vi "ClimberDeploy.vi"(8 "error in (no error)":errorcluster, 9 "Deploy":bool, 10 "Screw":dbl, 11 "Climber in":refnum<class "Climber.lvclass">) -> (0 "error out":errorcluster, 3 "Climber out":refnum<class "Climber.lvclass">)   [LabVIEW 2019, in "Climber.lvlib" / "Climber.lvclass"]
uses:
  Climber.lvclass
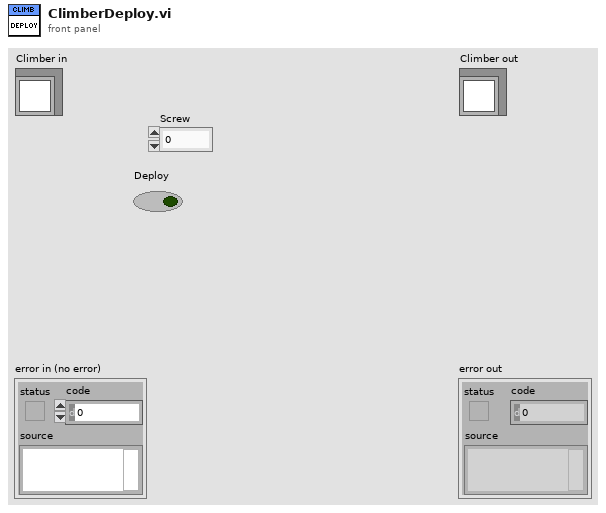
[diagram p1: front panel]
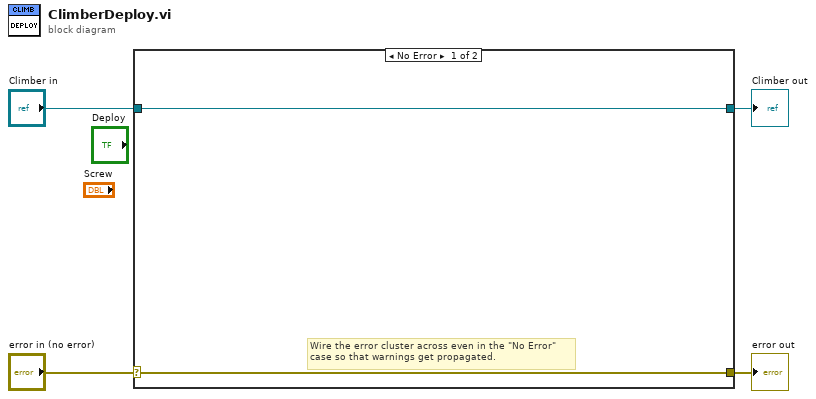
[diagram p0: block diagram]
diagram:
  n1 = case shown="No Error" "error in (no error)" {
    selector: "error in (no error)" -> [w5 w8]
    tunnel: [w5 w8] -> w3
    tunnel: [w6 w7] -> w1
    tunnel: "Climber in" -> [w6 w7]
    frame No Error {
      # "Wire the error cluster across even in the \"No Error\"\ncase so that warnings get propagated."
    }
    frame Error {
    }
  }
  "error out" <- w3
  "Climber out" <- w1
